vi "GetTimestampFpgaWithTach.vi"(4 "Enough Samples to Read":bool, 6 "Elements Remaining":u32, 7 "First Read":bool, 9 "Samples to Read":u32, 10 "Sampling Info":T1, 11 "Time Stamp in":timestamp) -> (3 "Time Stamp out":timestamp, 5 "adjusted time":bool)   [LabVIEW 2017, in "cRIOWfmLib.lvlib"]
uses:
  <vilib>/addons/InsightCM/Devices/Shared/Cms/cRIOWfmAcq/cRIOWfmLib.lvlib
  <vilib>/addons/InsightCM/Devices/Shared/Cms/cRIOWfmAcq/subVIs/RIO Wfm Cust Ctrls/rwfm_SamplingInfo.ctl
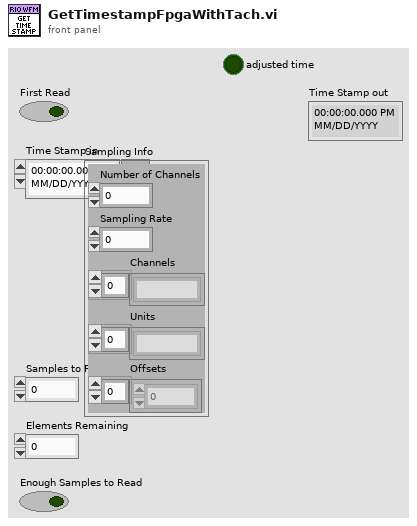
[diagram p1: front panel]
types:
  T1 = typedef "cRIOWfmLib.lvlib/rwfm_SamplingInfo.ctl" = cluster{"Number of Channels":i32, "Sampling Rate":dbl, "Channels":string[], "Units":string[], "Offsets":sgl[]}
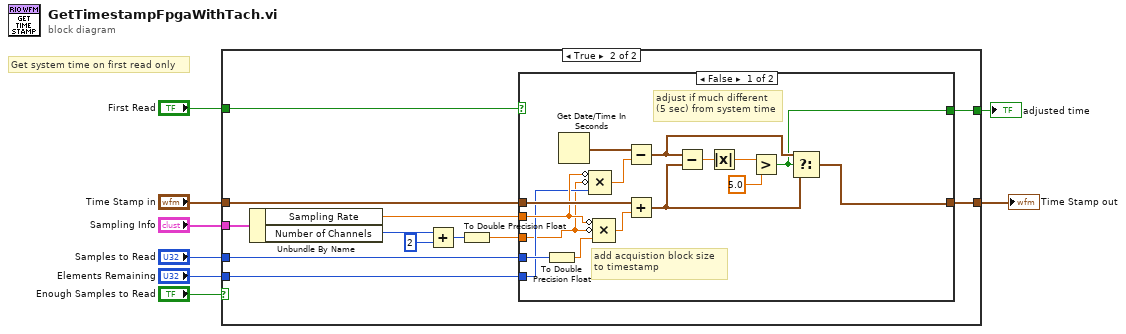
[diagram p0: block diagram]
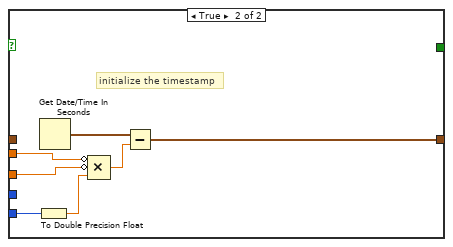
[diagram p3: hidden frame]
diagram:
  # "Get system time on first read only"
  n1 = case shown="True" "Enough Samples to Read" {
    tunnel: "Time Stamp in" -> [w9 w21]
    tunnel: "First Read" -> [_ w20]
    tunnel: "Sampling Info" -> [_ w18]
    tunnel: "Elements Remaining" -> [_ w17]
    tunnel: [w9 w16] -> w6
    tunnel: "Samples to Read" -> [_ w15]
    tunnel: [_ w10] -> w1
    frame False {
    }
    frame True {
      n2 = Unbundle By Name(w18) -> ("Sampling Rate"=w19:dbl, "Number of Channels"=w12:i32)
      n3 = Add(x=w12, y=2) -> (x+y=w13:i32)
      n4 = To Double Precision Float(number=w13) -> (double precision float=w14:dbl)
      n5 = case shown="False" w20 {
        tunnel: w19 -> [w28 w44]
        tunnel: w21 -> [w37 _]
        tunnel: w15 -> [w35 _]
        tunnel: w14 -> [w22 w43]
        tunnel: w17 -> [w27 w40]
        tunnel: [w31 w41] -> w16
        tunnel: [w23 _] -> w10
        frame False {
          # "adjust if much different (5 sec) from system time"
          # "add acquistion block size\nto timestamp"
          n6 = To Double Precision Float(number=w35) -> (double precision float=w34:dbl)
          n7 = Get Date/Time In Seconds() -> (seconds since 1Jan1904=w29:timestamp)
          n8 = Compound Arithmetic op=MULTIPLY(invert w28, invert w22, w27) -> (w30:dbl)
          n9 = Compound Arithmetic op=MULTIPLY(invert w28, invert w22, w34) -> (w36:dbl)
          n10 = Subtract(x=w29, y=w30) -> (x-y=w26:timestamp)
          n11 = Add(x=w37, y=w36) -> (x+y=w32:timestamp)
          n12 = Subtract(x=w26, y=w32) -> (x-y=w25:dbl)
          n13 = Absolute Value(x=w25) -> (abs(x)=w24:dbl)
          n14 = Greater?(x=w24, y=5.0) -> (0:w23:bool)
          n15 = Select(t=w26, s=w23, f=w32) -> (s? t:f=w31:timestamp)
        }
        frame True {
          # "initialize the timestamp"
          n16 = To Double Precision Float(number=w40) -> (double precision float=w39:dbl)
          n17 = Get Date/Time In Seconds() -> (seconds since 1Jan1904=w38:timestamp)
          n18 = Compound Arithmetic op=MULTIPLY(invert w44, invert w43, w39) -> (w42:dbl)
          n19 = Subtract(x=w38, y=w42) -> (x-y=w41:timestamp)
        }
      }
    }
  }
  "Time Stamp out" <- w6
  "adjusted time" <- w1
